vi "Time Estimate.vi"(8 "error in (no error)":errorcluster, 9 "expmode":i32, 10 "scantype":T1(ring), 11 "Wavelength Digikröm.lvclass":refnum<class "Wavelength Digikröm.lvclass">) -> (0 "error out":errorcluster, 1 "Time Estimate":string, 2 "time":dbl[unit], 3 "Wavelength Digikröm.lvclass":refnum<class "Wavelength Digikröm.lvclass">)   [LabVIEW 2012, in "Wavelength Digikröm.lvclass"]
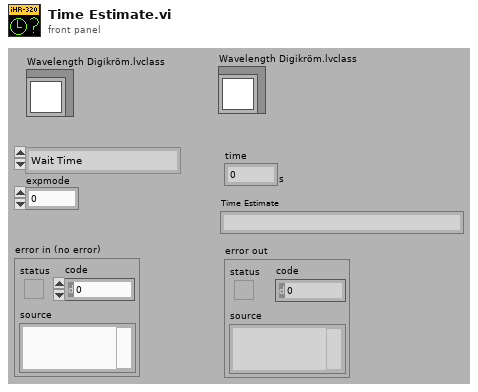
[diagram p1: front panel]
types:
  T1 = enum16{"Wait Time", "Pulse Width", "Wavelength", "Magnetic Field", "rf Scan"}
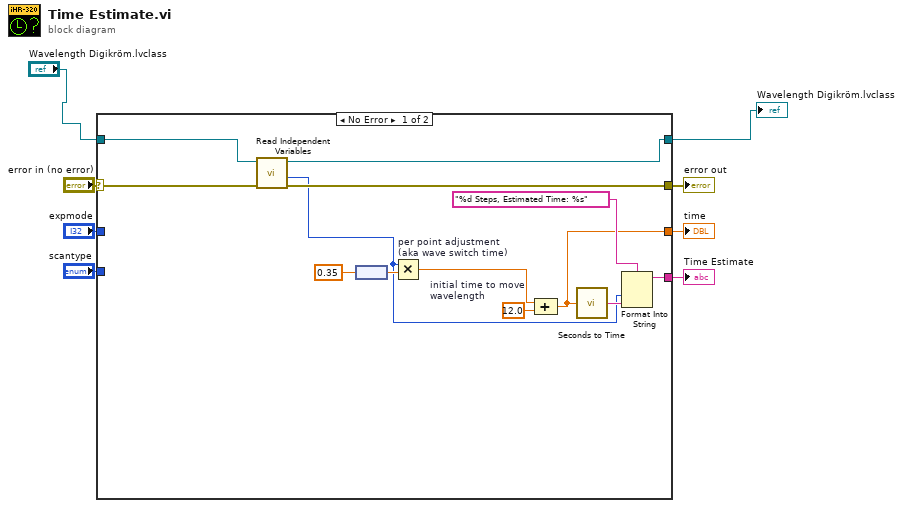
[diagram p0: block diagram]
diagram:
  n1 = case shown="No Error" "error in (no error)" {
    selector: "error in (no error)" -> [w18 w22]
    tunnel: [w14 _] -> w3
    tunnel: "expmode" -> [_ _]
    tunnel: "scantype" -> [_ _]
    tunnel: [w12 _] -> w6
    tunnel: [w19 w23] -> w2
    tunnel: "Wavelength Digikröm.lvclass" -> [w20 w23]
    tunnel: [w21 w22] -> w5
    frame No Error {
      w17 = dbl[unit] 12.0  # initial time to move wavelength
      n2 = call-dynamic "Read Independent Variables.vi"("error in (no error)"=w18, "Scanner.lvclass in"=w20) -> ("error out"=w21:errorcluster, "size"=w9:i32, "Scanner.lvclass out"=w19:refnum<class "Wavelength Digikröm.lvclass">)  [unwired: 7 out]
      n3 = node(0.35) -> (w10:dbl[unit])
      n4 = Multiply "per point adjustment\n(aka wave switch time)"(x=w9, y=w10) -> (x*y=w13:dbl[unit])
      n5 = Compound Arithmetic op=ADD(w13, w17) -> (w12:dbl[unit])
      n6 = call "Seconds to Time.vi"("Seconds"=w12) -> ("Time"=w15:string)
      n7 = Format Into String(format string="%d Steps, Estimated Time: %s", w9, w15) -> (resulting string=w14:string)  [unwired: 2 in, 1 out]
    }
    frame Error {
    }
  }
  "time" <- w6
  "error out" <- w5
  "Time Estimate" <- w3
  "Wavelength Digikröm.lvclass" <- w2
